vi "NT Read String Array.vi"(8 "error in":errorcluster, 9 "Default Value":string[](array[string]), 11 "Name":string="String Array") -> (0 "error out":errorcluster, 3 "String Array":string[](array[string]))   [LabVIEW 2017]
doc: "Return the string array data stored in the named entry. Return an error if not present or not a string array. Names that begin with a slash character \"/\" specify a full path, otherwise they are relative to /SmartDashboard/."
uses:
  <vilib>/Rock Robotics/Network Tables/Field Type.ctl
  <vilib>/Rock Robotics/Network Tables/Create Actual Table Name.vi
  <vilib>/Rock Robotics/Network Tables/Field Data Manager.vi
  <vilib>/Rock Robotics/Network Tables/Table Manager.vi
  <vilib>/Rock Robotics/Network Tables/Usage Statistics.vi
  <vilib>/Rock Robotics/Network Tables/NT Globals.vi
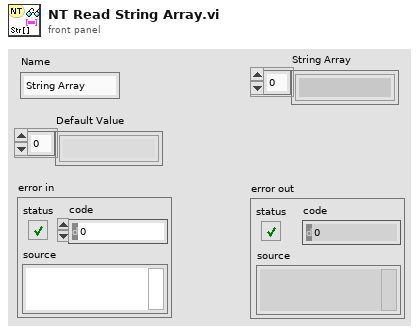
[diagram p1: front panel]
types:
  T1 = typedef "Field Type.ctl" = enum8{"Invalid", "Bool", "Numeric", "String", "Raw", "Boolean Array", "Numeric Array", "String Array", "RPC"}
  T2 = typedef "Field Data.ctl" = cluster{"Dbl":dbl, "String":string, "Type":T1, "Boolean":bool, "Sequence #":T3, "Flags":u8}
  T3 = typedef "Sequence.ctl" = u16
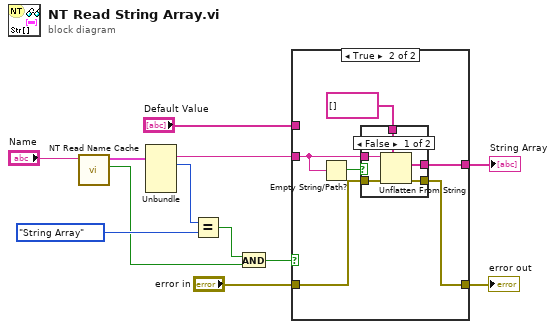
[diagram p0: block diagram]
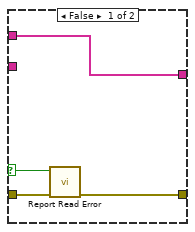
[diagram p2: hidden frame]
diagram:
  n1 = call <vilib>:"NT Read Name Cache.vi"("Name"="Name") -> ("Success"=w9:bool, "Field Value Out"=w8:T2)  [unwired: 9 in]
  n2 = Unbundle(w8) -> ("String"=w4:string, "Type"=w10:T1)  [unwired: 4 out]
  n3 = Equal?(x=w10, y=Field_Type."String Array" ("Type")) -> (x = y?=w12:bool)
  n4 = And(x=w12, y=w9) -> (x .and. y?=w5:bool)
  n5 = case shown="True" w5 {
    selector: w5 -> [w14 _]
    tunnel: [w16 w17] -> w1
    tunnel: "error in" -> [w15 w18]
    tunnel: w4 -> [_ w20]
    tunnel: "Default Value" -> [w13 _]
    tunnel: [w13 w19] -> w2
    frame False {
      n6 = call <vilib>:"Report Read Error.vi"("error in (no error)"=w15, "Success"=w14) -> ("error out"=w16:errorcluster)  [unwired: 9 in]
    }
    frame True {
      n7 = Empty String/Path?(string/path=w20) -> (empty?=w22:bool)
      n8 = case shown="False" w22 {
        tunnel: w20 -> [w27 _]
        tunnel: string[] [] ("Boolean Array") -> [w26 w29]
        tunnel: [w25 w29] -> w19
        tunnel: [w24 w28] -> w17
        tunnel: w18 -> [w23 w28]
        frame False {
          n9 = Unflatten From String(type=w26, binary string=w27, error in (no error)=w23) -> (value=w25:string[], error out=w24:errorcluster)  [unwired: 2 in, 1 out]
        }
        frame True {
        }
      }
    }
  }
  "String Array" <- w2
  "error out" <- w1
